vi "Assign Analog Inputs to Scope Channels.vi"(8 "error in (no error)":errorcluster, 11 "Program Data":T1 {"Time"."Time/Div" min=0.0 max=16.0 step=1.0 scale=0.0..12.0; "CH1"."Vertical Position (Div)" min=-5.0 max=5.0 step=0.1 scale=-5.0..5.0; "CH1"."Volts/Div" min=0 max=8 step=1 scale=0.0..8.0; "CH0"."Vertical Position (Div)" min=-5.0 max=5.0 step=0.1 scale=-5.0..5.0; "CH0"."Volts/Div" min=0 max=8 step=1 scale=0.0..8.0; "Wave Parameters"."Phase offset (deg)" format="%#_6p"; "Wave Parameters"."Frequency (Hz)" format="%#_6p"}) -> (0 "error out":errorcluster, 2 "Scope Data":waveform(dbl)[](array[waveform]), 3 "Program Data Out":T1 {"Time"."Time/Div" min=0.0 max=16.0 step=1.0 scale=0.0..12.0; "CH1"."Vertical Position (Div)" min=-5.0 max=5.0 step=0.1 scale=-5.0..5.0; "CH1"."Volts/Div" min=0 max=8 step=1 scale=0.0..8.0; "CH0"."Vertical Position (Div)" min=-5.0 max=5.0 step=0.1 scale=-5.0..5.0; "CH0"."Volts/Div" min=0 max=8 step=1 scale=0.0..8.0; "Wave Parameters"."Phase offset (deg)" format="%#_6p"; "Wave Parameters"."Frequency (Hz)" format="%#_6p"})   [LabVIEW 2021]
uses:
  Controls/Program Data.ctl
  Controls/Measurements.ctl
  Controls/Channel Measurement String Control.ctl
  Controls/Cursor Info.ctl
  Controls/Communication Cluster.ctl
  <vilib>/NI/STM/TCP/TCP Connection Info.ctl
  <vilib>/NI/STM/SubVIs/MetaDataElement.ctl
  Communication/Scope Data.ctl
  Program Files (x86)/National Instruments/LabVIEW 2021/ProjectTemplates/Source/myRIO/Oscilloscope/myRIO v1.1/Real-Time/Controls/Wave Parameters.ctl
  Program Files (x86)/National Instruments/LabVIEW 2021/ProjectTemplates/Source/myRIO/Oscilloscope/myRIO v1.1/Real-Time/Controls/Waveform Enum.ctl
  Program Files (x86)/National Instruments/LabVIEW 2021/ProjectTemplates/Source/myRIO/Oscilloscope/myRIO v1.1/Real-Time/Controls/Channel Selector.ctl
  Controls/Channel Settings.ctl
  Controls/Analog Input Selector.ctl
  Controls/Knob.ctl
  Controls/Vertical Position.ctl
  Controls/Channel Parameters.ctl
  Controls/Time Selector.ctl
  Controls/Time Knob.ctl
  Controls/FGen Desktop Configuration.ctl
  <vilib>/NI/STM/NI STM.lvlib
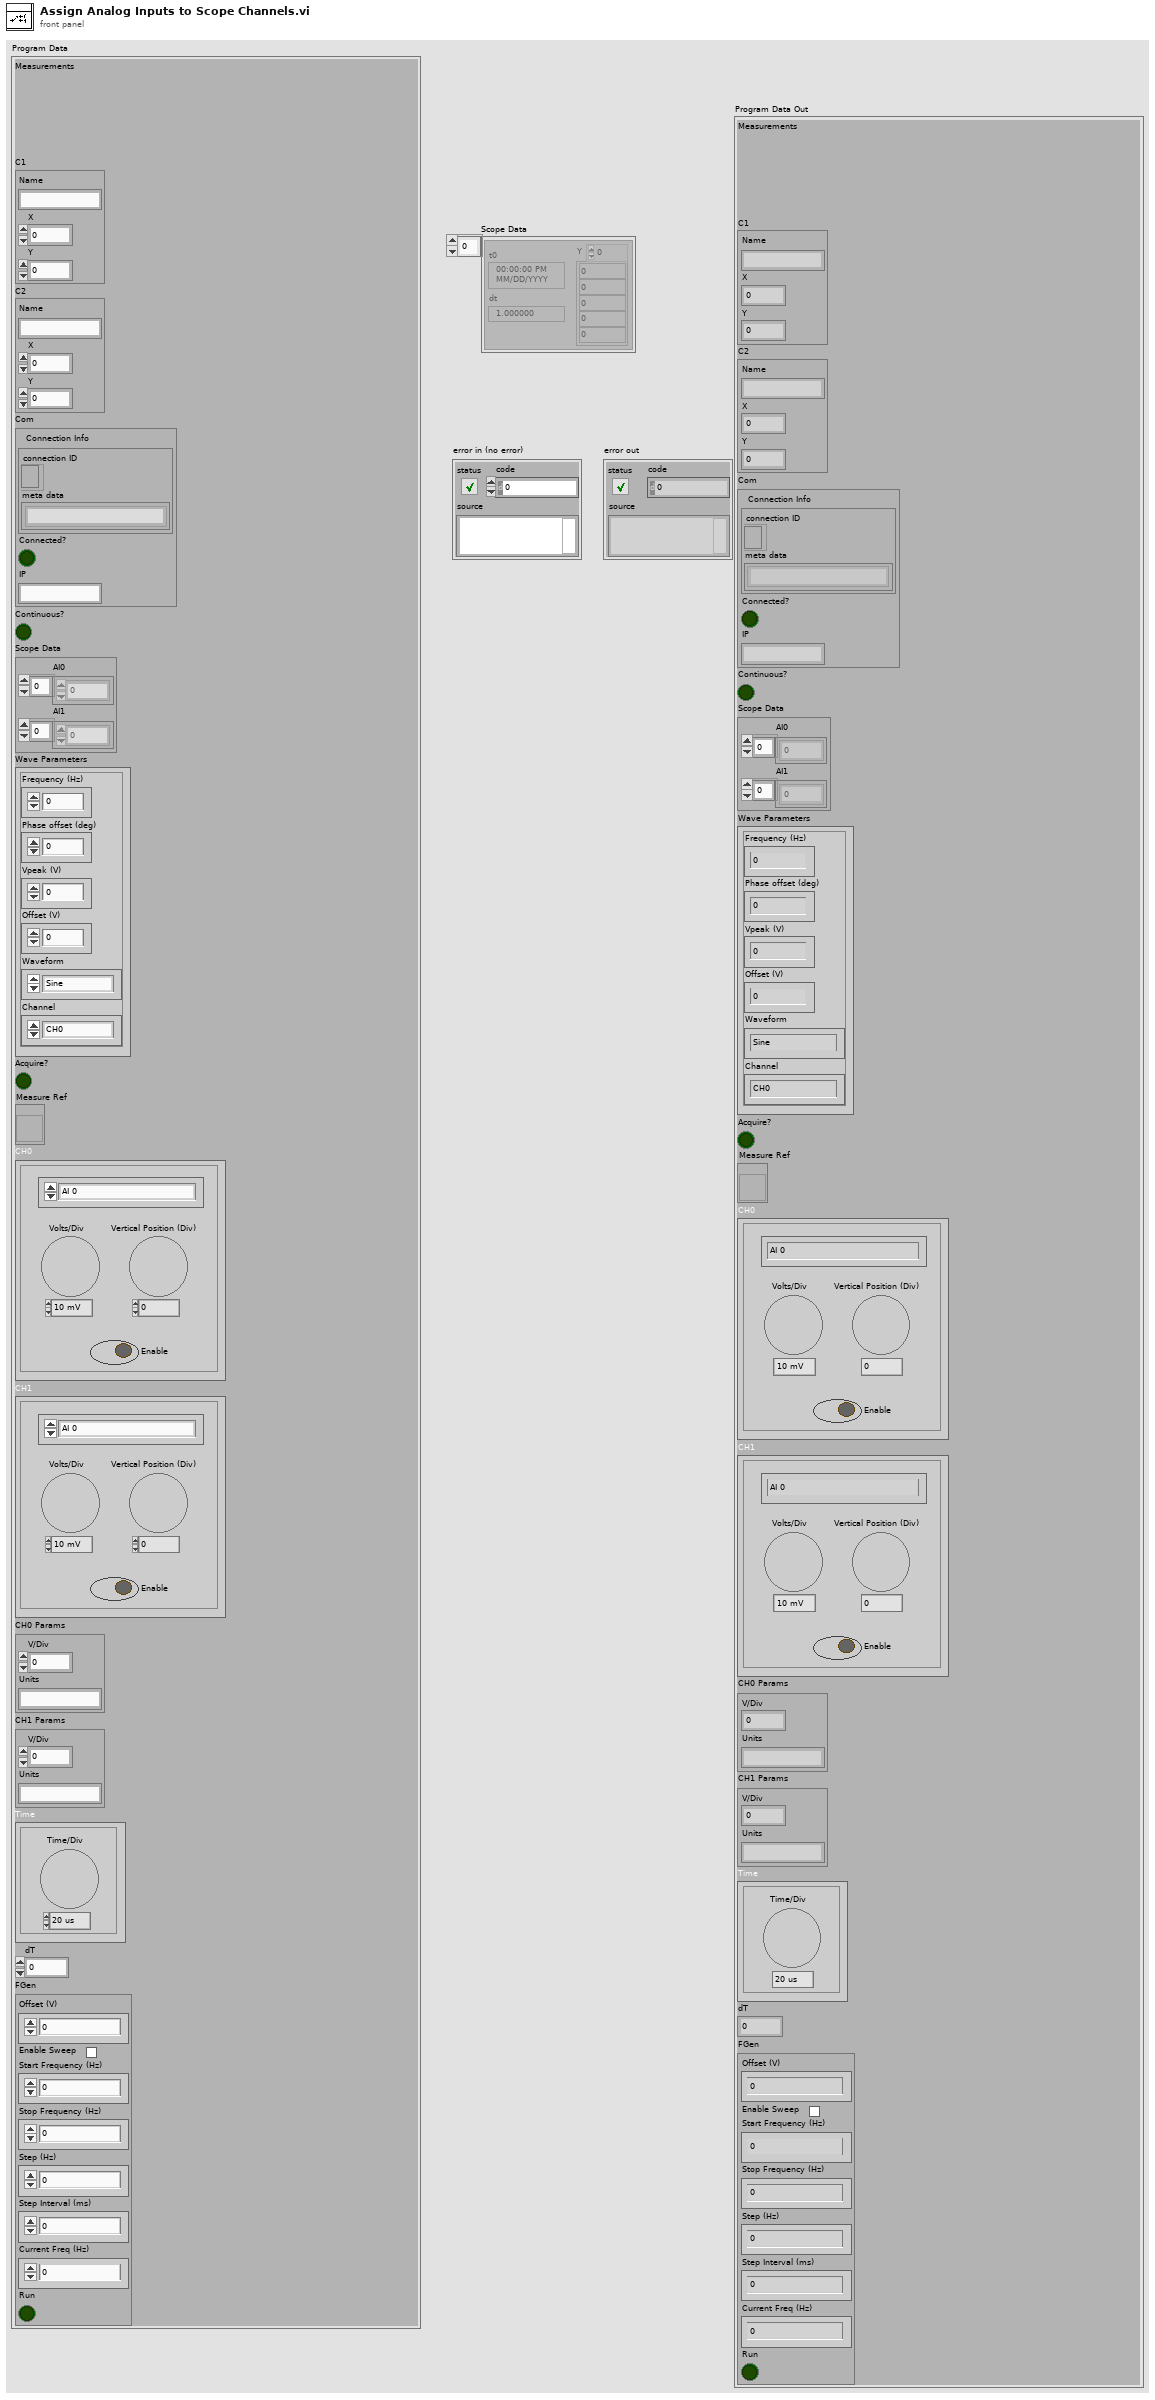
[diagram p1: front panel]
types:
  T1 = typedef "Program Data.ctl" = cluster{"Measurements":T2, "C1":T4, "C2":T4, "Com":T5, "Continuous?":bool, "Scope Data":T8, "Wave Parameters":T9, "Acquire?":bool, "Measure Ref":refnum<vi>, "CH0":T12, "CH1":T12, "CH0 Params":T16, "CH1 Params":T16, "Time":T17, "dT":dbl, "FGen":T19}
  T2 = typedef "Measurements.ctl" = cluster{"Channel 0":T3, "RMS 0":T3, "Vp-p 0":T3, "Freq 0":T3, "Channel 1":T3, "RMS 1":T3, "Vp-p 1":T3, "Freq 1":T3, "Cursors":T3, "C1":T3, "C2":T3, "dT":T3}
  T3 = typedef "Channel Measurement String Control.ctl" = string
  T4 = typedef "Cursor Info.ctl" = cluster{"Name":string, "X":dbl, "Y":dbl}
  T5 = typedef "Communication Cluster.ctl" = cluster{"Connection Info":T6, "Connected?":bool, "IP":string}
  T6 = typedef "NI STM.lvlib/TCP Connection Info.ctl" = cluster{"connection ID":refnum<k5>, "meta data":T7[]}
  T7 = typedef "NI STM.lvlib/MetaDataElement.ctl" = string
  T8 = typedef "Scope Data.ctl" = cluster{"AI0":dbl[], "AI1":dbl[]}
  T9 = typedef "Wave Parameters.ctl" = cluster{"Frequency (Hz)":dbl, "Phase offset (deg)":dbl, "Vpeak (V)":dbl, "Offset (V)":dbl, "Waveform":T10, "Channel":T11}
  T10 = typedef "Waveform Enum.ctl" = enum16{"Sine", "Square"}
  T11 = typedef "Channel Selector.ctl" = enum16{"CH0", "CH1"}
  T12 = typedef "Channel Settings.ctl" = cluster{"Channel":T13, "Enable":bool, "Volts/Div":T14, "Vertical Position (Div)":T15}
  T13 = typedef "Analog Input Selector.ctl" = enum16{"AI 0", "AI 1"}
  T14 = typedef "Knob.ctl" = i32
  T15 = typedef "Vertical Position.ctl" = dbl
  T16 = typedef "Channel Parameters.ctl" = cluster{"V/Div":dbl, "Units":string}
  T17 = typedef "Time Selector.ctl" = cluster{"Time/Div":T18}
  T18 = typedef "Time Knob.ctl" = dbl
  T19 = typedef "FGen Desktop Configuration.ctl" = cluster{"Offset (V)":dbl, "Enable Sweep":bool, "Start Frequency (Hz)":dbl, "Stop Frequency (Hz)":dbl, "Step (Hz)":dbl, "Step Interval (ms)":dbl, "Current Freq (Hz)":dbl, "Run":bool}
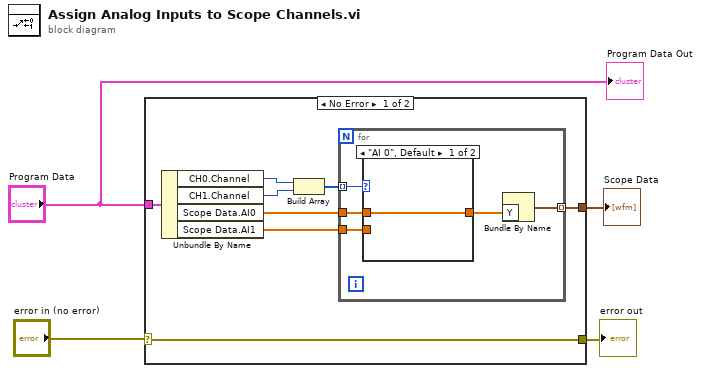
[diagram p0: block diagram]
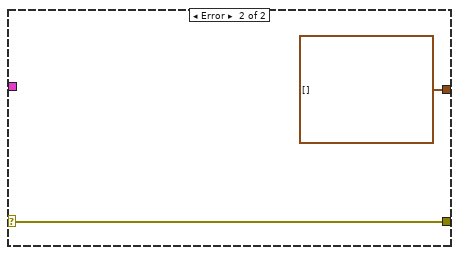
[diagram p3: hidden frame]
diagram:
  n1 = case shown="No Error" "error in (no error)" {
    selector: "error in (no error)" -> [w5 w21]
    tunnel: "Program Data" -> [w12 _]
    tunnel: [w6 waveform(dbl)[] []] -> w3
    tunnel: [w5 w21] -> w1
    frame No Error {
      n2 = Unbundle By Name(w12) -> ("CH0.Channel"=w11:T13, "CH1.Channel"=w10:T13, "Scope Data.AI0"=w8:dbl[], "Scope Data.AI1"=w7:dbl[])
      n3 = Build Array(w11, w10) -> (w9:T13[])
      n4 = for {
        tunnel: w9 -> [w17] mode=indexing
        tunnel: w8 -> [w16]
        tunnel: w7 -> [w15]
        tunnel: [w13] -> w6 mode=indexing
        n5 = case shown="\"AI 0\", Default" w17 {
          tunnel: w16 -> [w18 _]
          tunnel: w15 -> [_ w19]
          tunnel: [w18 w19] -> w14
          frame "AI 0", Default {
          }
          frame "AI 1" {
          }
        }
        n6 = Bundle By Name("Y"=w14) -> (w13:waveform(dbl))  [unwired: 1 in]
      }
    }
    frame Error {
    }
  }
  "Scope Data" <- w3
  "error out" <- w1
  "Program Data Out" <- "Program Data"
